vi "Disable Debugging for all VIs in Project.vi"   [LabVIEW 2025]
uses:
  <vilib>/Utility/EditLVProj/Edit LVProj.lvlib
types:
  T1 = typedef "Edit LVProj.lvlib/Library And VI References.ctl" = cluster{"Target Reference":refnum<vi>, "VI References":refnum<vi>[], "Library References":refnum<vi>[]}
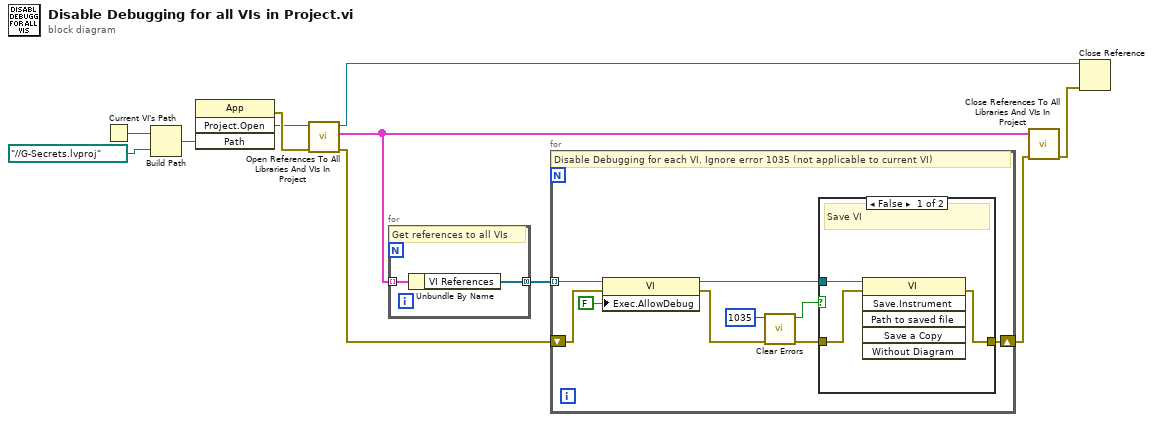
[diagram p0: block diagram]
diagram:
  n1 = Current VI's Path() -> (path=w3:path)
  n2 = Build Path(base path=w3, name or relative path=path "../../G-Secrets.lvproj" ("Path")) -> (appended path=w1:path)
  n3 = invoke class="App" method="Project.Open"("Path"=w1) -> (error out=w11:errorcluster, "Project:Open"=w6:refnum<vi>)  [unwired: 3 in, 2 out]
  n4 = call <vilib>:"Open References To All Libraries And VIs In Project.vi"("error in (no error)"=w11, "Project in"=w6) -> ("error out"=w10:errorcluster, "VI and Library References"=w5:T1[], "Project out"=w4:refnum<vi>)  [unwired: 7 in]
  n5 = for {
    tunnel: w5 -> [w13] mode=indexing
    tunnel: [w12] -> w7 mode=concatenating
    # "Get references to all VIs"
    n6 = Unbundle By Name(w13) -> ("VI References"=w12:refnum<vi>[])
  }
  n7 = for {
    tunnel: w7 -> [w18] mode=indexing
    shift-right: [w21] -> w9
    shift-left: w10 -> [w22]
    # "Disable Debugging for each VI. Ignore error 1035 (not applicable to current VI)"
    n8 = property class="VI"(reference=w18, error in=w22, "Exec.AllowDebug"=FALSE ("Execution:Allow Debugging")) -> (reference out=w16:refnum<vi>, error out=w20:errorcluster)
    n9 = call <vilib>:"Clear Errors.vi"("error in (no error)"=w20, "specific error code to clear (0: all)"=1035) -> ("error out"=w19:errorcluster, "specific error cleared?"=w14:bool)  [unwired: 4 in]
    n10 = case shown="False" w14 {
      tunnel: w16 -> [w23 _]
      tunnel: [w25 w26] -> w21
      tunnel: w19 -> [w24 w26]
      frame False {
        # "Save VI"
        n11 = invoke class="VI" method="Save.Instrument"(reference=w23, error in=w24) -> (error out=w25:errorcluster)  [unwired: 4 in, 5 out]
      }
      frame True {
        # "Error occurred, do not save"
      }
    }
  }
  n12 = call <vilib>:"Close References To All Libraries And VIs In Project.vi"("error in (no error)"=w9, "VI and Library References"=w5) -> ("error out"=w8:errorcluster)  [unwired: 9 in]
  n13 = Close Reference(reference=w4, error in (no error)=w8) -> ()  [unwired: 1 out]
